vi "Get Fixture Object.vi"(6 "Gantry map":dbl[](array[numeric]), 8 "error in (no error)":errorcluster, 9 "Routine":T1=enum."Dispense on Plate", 10 "Module In":refnum<class "Module.lvclass">, 11 "Fixture":T2) -> (0 "error out":errorcluster, 2 "Module Out":refnum<class "Module.lvclass">, 3 "Workspace.lvclass":refnum<class "Fixture.lvclass">)   [LabVIEW 2021, in "Fixture.lvclass"]
uses:
  Fixture.lvclass
  Fixture Enum.ctl
  Module/Module.lvclass
  Routine/Routine Enum.ctl
  Carrier Tray/Assembly Tray.lvclass
  C:/Users/hep/Documents/UCSB-CMU-GantryCode/UCSB-Gantry-HEP-main (3)/UCSB-Gantry-HEP-main/Classes/Workspace/Fixture.lvclass
  Component/Component Tray.lvclass
  Pick Up Tool Area/Pick Up Tool Fixture.lvclass
  In Place/Current Position.lvclass
  Carrier Tray/Syringe Space/Syringe Space.lvclass
  Module/Read Instantiated.vi
  Routine/Routine.lvclass
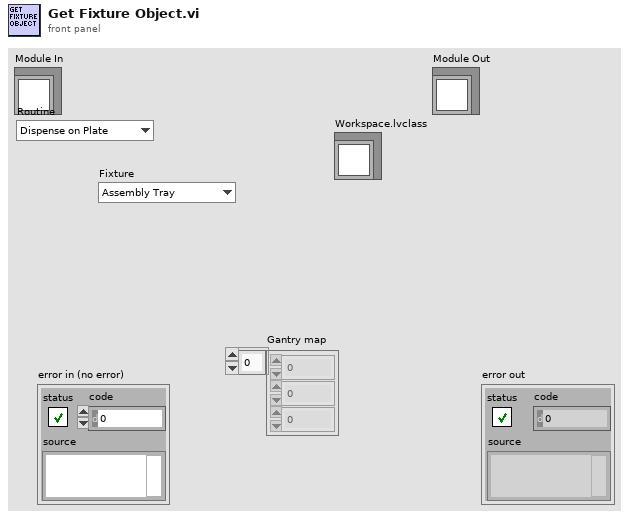
[diagram p1: front panel]
types:
  T1 = typedef "Routine.lvclass/Routine Enum.ctl" = enum16{"Primary Pick Up", "Secondary Pick Up", "Put Down All", "Secure Syringe", "Release Syringe", "Dispense on Plate", "Dispense on Sensor", "Pick Up All", "Put Down Secondary", "Dispense on Kapton"}
  T2 = typedef "Fixture.lvclass/Fixture Enum.ctl" = enum16{"Assembly Tray", "Syringe Space", "Component", "Pick Up Tool", "Current Position"}
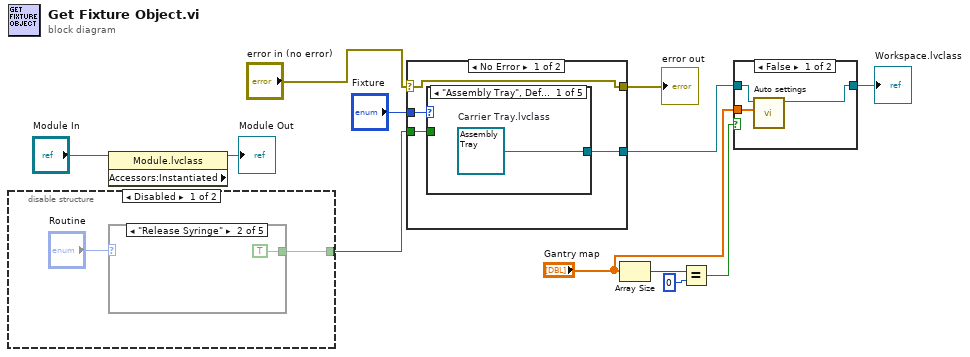
[diagram p0: block diagram]
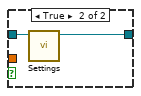
[diagram p2: hidden frame]
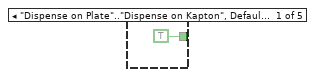
[diagram p3: hidden frame]
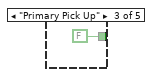
[diagram p4: hidden frame]
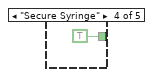
[diagram p5: hidden frame]
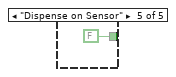
[diagram p6: hidden frame]
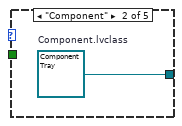
[diagram p8: hidden frame]
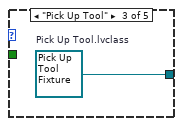
[diagram p9: hidden frame]
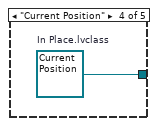
[diagram p10: hidden frame]
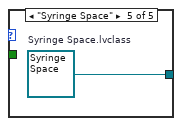
[diagram p11: hidden frame]
diagram:
  n1 = disable-structure shown="Disabled" {
    disable-tunnel: [w13 _] -> w5
    frame Disabled {
      n2 = case shown="\"Release Syringe\"" "Routine" {
        tunnel: [TRUE TRUE FALSE TRUE FALSE] -> w13
        frame "Dispense on Plate".."Dispense on Kapton", Default {
        }
        frame "Release Syringe" {
        }
        frame "Primary Pick Up" {
        }
        frame "Secure Syringe" {
        }
        frame "Dispense on Sensor" {
        }
      }
    }
    frame Enabled {
    }
  }
  n3 = property class="Module.lvclass" props=["Accessors:Instantiated"](reference="Module In") -> (reference out=→"Module Out":refnum<class "Module.lvclass">)  [unwired: 1 in, 2 out]
  n4 = case shown="No Error" "error in (no error)" {
    selector: "error in (no error)" -> [w21 w29]
    tunnel: [w21 w29] -> w11
    tunnel: "Fixture" -> [w23 _]
    tunnel: [w22 _] -> w9
    tunnel: w5 -> [w20 _]
    frame No Error {
      n5 = case shown="\"Assembly Tray\", Default" w23 {
        tunnel: [w24 w25 w26 w27 w28] -> w22
        tunnel: w20 -> [_ _ _ _ _]
        frame "Assembly Tray", Default {
          w24 = refnum<class "Assembly Tray.lvclass"> refnum  # Carrier Tray.lvclass
        }
        frame "Component" {
          w25 = refnum<class "Component Tray.lvclass"> refnum  # Component.lvclass
        }
        frame "Pick Up Tool" {
          w26 = refnum<class "Pick Up Tool Fixture.lvclass"> refnum  # Pick Up Tool.lvclass
        }
        frame "Current Position" {
          w27 = refnum<class "Current Position.lvclass"> refnum  # In Place.lvclass
        }
        frame "Syringe Space" {
          w28 = refnum<class "Syringe Space.lvclass"> refnum  # Syringe Space.lvclass
        }
      }
    }
    frame Error {
    }
  }
  "error out" <- w11
  n6 = Array Size(array="Gantry map") -> (size(s)=w3:i32)
  n7 = Equal?(x=w3, y=0) -> (x = y?=w2:bool)
  n8 = case shown="False" w2 {
    tunnel: w9 -> [w30 w34]
    tunnel: [w31 w33] -> w8
    tunnel: "Gantry map" -> [w32 _]
    frame False {
      n9 = call-dynamic "Auto settings.vi"("Array"=w32, "Fixture in"=w30) -> ("Fixture out"=w31:refnum<class "Fixture.lvclass">)  [unwired: 8 in, 1 out]
    }
    frame True {
      n10 = call-dynamic "Settings.vi"("Workspace in"=w34) -> ("Workspace out"=w33:refnum<class "Fixture.lvclass">)  [unwired: 9 in, 1 out]
    }
  }
  "Workspace.lvclass" <- w8
